vi "Re_Initialisation_Counter.vi"() -> ()   [LabVIEW 2012]
panel:
  in  "Re-initialisation counter":u32
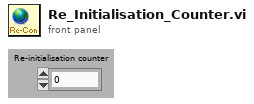
[diagram p1: front panel]
diagram:
